vi "CAEN PSM Output DC Volts.vi"() -> ()   [LabVIEW 2018]
doc: "This example shows how to configure the instrument's output voltage level, over current protection, and over voltage protection. The actual voltage level and actual current level are returned as well as whether over voltage protection (OVP) or over current protection (OCP) has been tripped."
uses:
  <instrlib>/CAEN PSM/CAEN PSM.lvlib
panel:
  in  "Stop Output":bool
  out "OVC?":bool
  out "OVV?":bool
  in  "Voltage Max (0V)":dbl format="%.2f"
  out "Actual Current Limit (uA)":dbl format="%.2f"
  out "Actual Voltage Level (V)":dbl format="%.2f"
  in  "Voltage Level (0.0 V)":dbl format="%.2f"
  in  "Current Limit (0 uA)":dbl format="%.2f"
  in  "Channel":u8(ring) items=["Channel 0", "Channel 1", "Channel 2", "Channel 3"]
  in  "VISA resource name":refnum<visa-resource-name>
  # "(c) 2012 CAEN SpA.  ALL RIGHTS RESERVED."
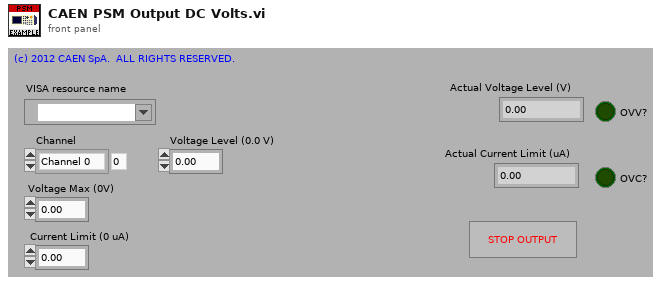
[diagram p1: front panel]
types:
  T1 = typedef "CAEN PSM.lvlib/BoardHandle.ctl" = cluster{"VISA resource name":refnum<visa-resource-name>, "Board address":u8, "NChannels":u8}
  T2 = cluster{"ON":bool, "RUP":bool, "RDW":bool, "OVC":bool, "OVV":bool, "UNV":bool, "MAXV":bool, "TRIP":bool, "OVP":bool, "OVT":bool, "DIS":bool, "KILL":bool, "ILK":bool, "NOCAL":bool}[]
  T3 = cluster{"ON":bool, "RUP":bool, "RDW":bool, "OVC":bool, "OVV":bool, "UNV":bool, "MAXV":bool, "TRIP":bool, "OVP":bool, "OVT":bool, "DIS":bool, "KILL":bool, "ILK":bool, "NOCAL":bool}
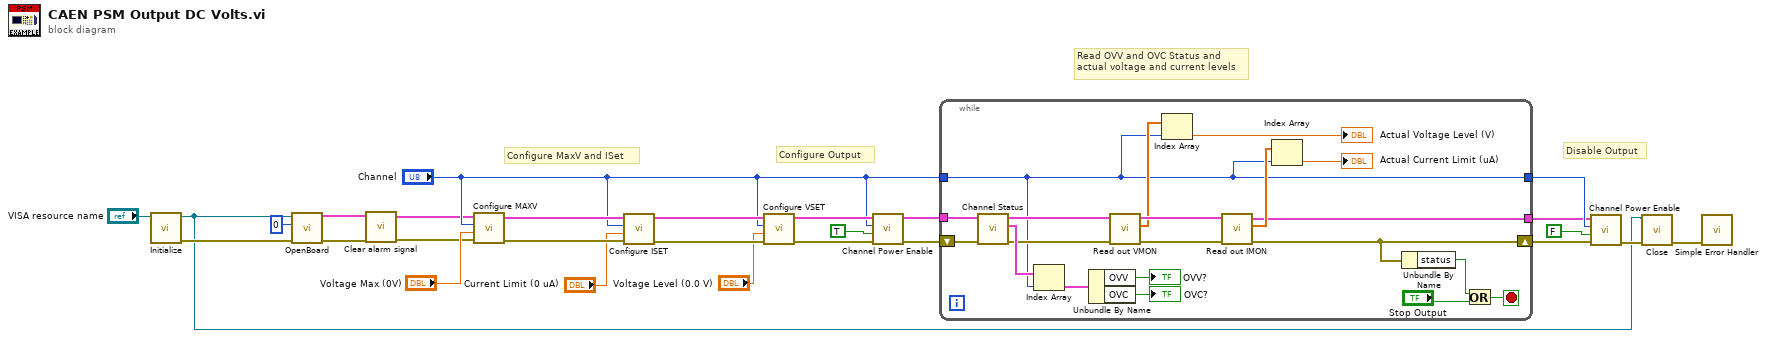
[diagram p0: block diagram]
diagram:
  # "Disable Output"
  # "Read OVV and OVC Status and\nactual voltage and current levels"
  # "Configure Output"
  # "Configure MaxV and ISet"
  n1 = call <instrlib>:"Initialize.vi"("VISA resource name"="VISA resource name") -> ("error out"=w19:errorcluster, "VISA resource name out"=w6:refnum<visa-resource-name>)  [unwired: 9 in]
  n2 = call <instrlib>:"OpenBoard.vi"("error in (no error)"=w19, "Board Address"=u8 0, "VISA resource name"=w6) -> ("error out"=w4:errorcluster, "BoardHandle"=w1:T1)  [unwired: 7 in]
  n3 = call <instrlib>:"Clear alarm signal.vi"("error in (no error)"=w4, "BoardHandle"=w1) -> ("error out"=w3:errorcluster, "BoardHandle out"=w2:T1)  [unwired: 8 in]
  n4 = call <instrlib>:"Configure MAXV.vi"("error in (no error)"=w3, "Voltage Max (0.0 V)"="Voltage Max (0V)", "Channel (0)"="Channel", "BoardHandle"=w2) -> ("error out"=w22:errorcluster, "BoardHandle out"=w17:T1)  [unwired: 6 in]
  n5 = call <instrlib>:"Configure ISET.vi"("error in (no error)"=w22, "Current Limit (0.00 uA)"="Current Limit (0 uA)", "Channel (0)"="Channel", "BoardHandle"=w17) -> ("error out"=w26:errorcluster, "BoardHandle out"=w15:T1)  [unwired: 6 in]
  n6 = call <instrlib>:"Configure VSET.vi"("error in (no error)"=w26, "Voltage Level (0.0 V)"="Voltage Level (0.0 V)", "Channel (0)"="Channel", "BoardHandle"=w15) -> ("error out"=w14:errorcluster, "BoardHandle out"=w11:T1)  [unwired: 6 in]
  n7 = call <instrlib>:"Channel Power Enable.vi"("error in (no error)"=w14, "Enable (OFF)"=TRUE, "Channel (0)"="Channel", "BoardHandle"=w11) -> ("error out"=w13:errorcluster, "BoardHandle out"=w12:T1)  [unwired: 6 in]
  n8 = while {
    tunnel: w12 -> [w47]
    tunnel: "Channel" -> [w28]
    tunnel: [w28] -> w20
    shift-right: [w34] -> w24
    shift-left: w13 -> [w46]
    tunnel: [w29] -> w5
    stop <- w45 stop-if-true
    n9 = call <instrlib>:"Channel Status.vi"("error in (no error)"=w46, "BoardHandle"=w47) -> ("error out"=w38:errorcluster, "Channel Status Array"=w42:T2, "BoardHandle out"=w37:T1)  [unwired: 7 in]
    n10 = Index Array(array=w42, index=w28) -> (element=w41:T3)
    n11 = Unbundle By Name(w41) -> ("OVV"=→"OVV?":bool, "OVC"=→"OVC?":bool)
    n12 = call <instrlib>:"Read out VMON.vi"("error in (no error)"=w38, "BoardHandle"=w37) -> ("error out"=w35:errorcluster, "VMon values (V)"=w33:dbl[], "BoardHandle out"=w36:T1)  [unwired: 7 in]
    n13 = Index Array(array=w33, index=w28) -> (element=→"Actual Voltage Level (V)":dbl)
    n14 = call <instrlib>:"Read out IMON.vi"("error in (no error)"=w35, "BoardHandle"=w36) -> ("error out"=w34:errorcluster, "IMon values (uA)"=w30:dbl[], "BoardHandle out"=w29:T1)  [unwired: 6 in, 1 out]
    n15 = Index Array(array=w30, index=w28) -> (element=→"Actual Current Limit (uA)":dbl)
    n16 = Unbundle By Name(w34) -> ("status"=w43:bool)
    n17 = Or(x=w43, y="Stop Output") -> (x .or. y?=w45:bool)
  }
  n18 = call <instrlib>:"Channel Power Enable.vi"("error in (no error)"=w24, "Enable (OFF)"=FALSE, "Channel (0)"=w20, "BoardHandle"=w5) -> ("error out"=w23:errorcluster)  [unwired: 6 in, 1 out]
  n19 = call <instrlib>:"Close.vi"("error in (no error)"=w23, "VISA resource name"=w6) -> ("error out"=w8:errorcluster)  [unwired: 9 in]
  n20 = call <vilib>:"Simple Error Handler.vi"("error in (no error)"=w8) -> ()  [unwired: 4 in, 5 out]
